vi "Test Action Global.vi"(7 "Write (F)":bool, 10 "Data IN":dbl format="%#_13g", 11 "Test Action IN":T1=enum."Start") -> (2 "Data OUT":dbl, 3 "Test Action OUT":T1=enum."Start")   [LabVIEW 2019]
uses:
  Controls/Test Action.ctl
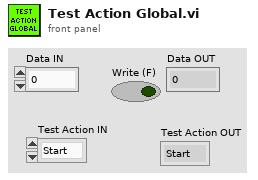
[diagram p1: front panel]
types:
  T1 = typedef "Test Action.ctl" = enum16{"Idle", "Start", "Stop", "Pump Cmd", "Pump 1 Enable", "Pump 2 Enable", "Pump 3 Enable", "Pump 4 Enable", "Pump 5 Enable", "Pump 6 Enable", "Timer 1 Reset", "Timer 2 Reset", "Timer 3 Reset", "Timer 4 Reset", "Timer 5 Reset", "Timer 6 Reset"}
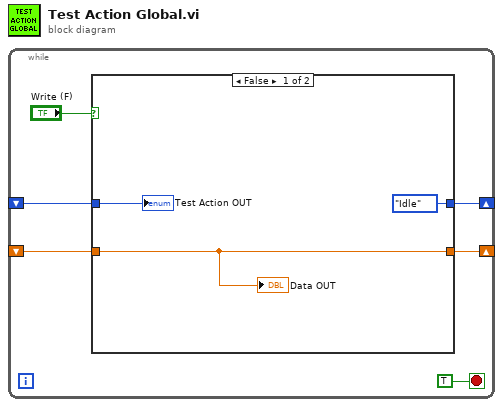
[diagram p0: block diagram]
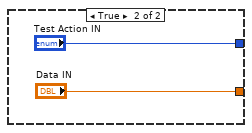
[diagram p2: hidden frame]
diagram:
  n1 = while {
    shift-right: [w4] -> _
    shift-left: _ -> [w3]
    shift-right: [w2] -> _
    shift-left: _ -> [w1]
    stop <- TRUE stop-if-true
    n2 = case shown="False" "Write (F)" {
      tunnel: [Test_Action."Idle" ("Test Action IN") "Test Action IN"] -> w4
      tunnel: w3 -> [w9 _]
      tunnel: [w7 "Data IN"] -> w2
      tunnel: w1 -> [w7 _]
      frame False {
        "Test Action OUT" <- w9
        "Data OUT" <- w7
      }
      frame True {
      }
    }
  }
